vi "MotionMacro@CombineMotion__Parameter.vi"(1 "ParamterIn":string) -> (0 "ParamterOut":string)   [LabVIEW 2020]
panel:
  in  "AxisU":string(combo)
  in  "AxisZ":string(combo)
  in  "AxisY":string(combo)
  in  "AxisX":string(combo)
  in  "CombineMotor":string(combo)
  in  "Confirm":bool
  # "MotorMacro@CombineMotion $CombinName,$AxisX,$AxisY(,$AxisZ.....)"
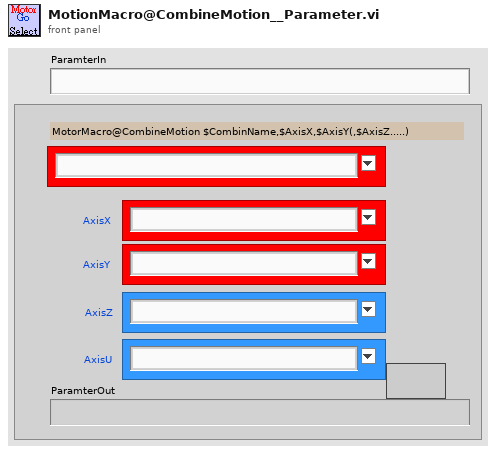
[diagram p1: front panel]
types:
  T1 = enum16{"Get", "Init", "Set", "Delete", "GetElement", "Inc", "Dec", "ReName", "Copy"}
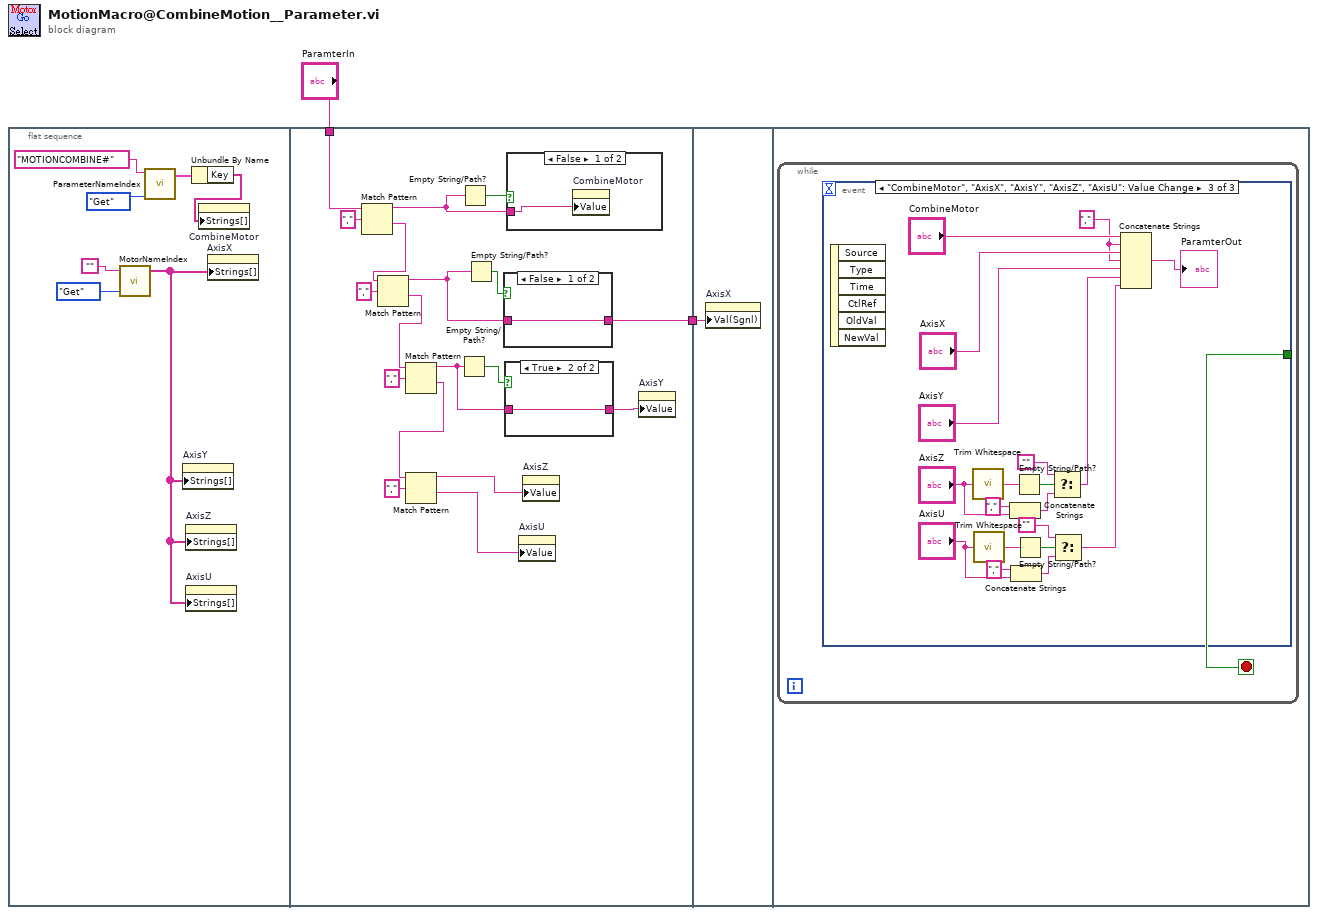
[diagram p0: block diagram]
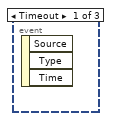
[diagram p5: hidden frame]
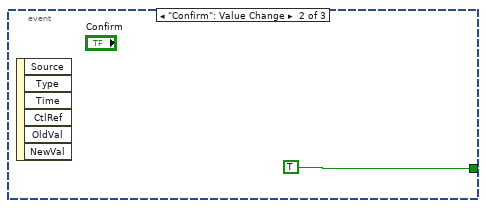
[diagram p6: hidden frame]
diagram:
  n1 = flat-sequence {
    tunnel: "ParamterIn" -> [w24]
    tunnel: [w25] -> w1
    tunnel: w1 -> [w33]
    frame #0 {
      n2 = call "MotorNameIndex.vi"("OP"=enum16{"Get", "Update", "Init"}."Get", "MotorName"="") -> ("MotorList"=w7:string[])  [unwired: 1 in, 2 out]
      n3 = call "ParameterNameIndex.vi"("OP"=T1."Get", "VariableSection"="MOTIONCOMBINE#" ("string")) -> ("SectionKeyValue"=w4:cluster{"Key":string[], "Value":string[]})  [unwired: 3 in, 6 out]
      n4 = property on="AxisY" class="CmbBox"("Strings[]"=w7) -> ()  [unwired: 2 in, 2 out]
      n5 = property on="AxisZ" class="CmbBox"("Strings[]"=w7) -> ()  [unwired: 2 in, 2 out]
      n6 = property on="AxisU" class="CmbBox"("Strings[]"=w7) -> ()  [unwired: 2 in, 2 out]
      n7 = Unbundle By Name(w4) -> ("Key"=w3:string[])
      n8 = property on="CombineMotor" class="CmbBox"("Strings[]"=w3) -> ()  [unwired: 2 in, 2 out]
      n9 = property on="AxisX" class="CmbBox"("Strings[]"=w7) -> ()  [unwired: 2 in, 2 out]
    }
    frame #1 {
      n10 = Match Pattern(string=w24, regular expression="," ("search string")) -> (before substring=w22:string, after substring=w20:string)  [unwired: 1 in, 2 out]
      n11 = Match Pattern(string=w20, regular expression="," ("search string")) -> (before substring=w19:string, after substring=w17:string)  [unwired: 1 in, 2 out]
      n12 = Match Pattern(string=w17, regular expression="," ("search string")) -> (before substring=w14:string, after substring=w12:string)  [unwired: 1 in, 2 out]
      n13 = Match Pattern(string=w12, regular expression="," ("search string")) -> (before substring=w11:string, after substring=w10:string)  [unwired: 1 in, 2 out]
      n14 = Empty String/Path?(string/path=w14) -> (empty?=w16:bool)
      n15 = Empty String/Path?(string/path=w22) -> (empty?=w27:bool)
      n16 = Empty String/Path?(string/path=w19) -> (empty?=w26:bool)
      n17 = case shown="False" w26 {
        tunnel: [w30 w31] -> w25
        tunnel: w19 -> [w30 w31]
        frame False {
        }
        frame True {
        }
      }
      n18 = case shown="True" w16 {
        tunnel: [w28 w29] -> w15
        tunnel: w14 -> [w28 w29]
        frame False {
        }
        frame True {
        }
      }
      n19 = case shown="False" w27 {
        tunnel: w22 -> [w32 _]
        frame False {
          n20 = property on="CombineMotor" class="CmbBox"("Value"=w32) -> ()  [unwired: 2 in, 2 out]
        }
        frame True {
        }
      }
      n21 = property on="AxisU" class="CmbBox"("Value"=w10) -> ()  [unwired: 2 in, 2 out]
      n22 = property on="AxisZ" class="CmbBox"("Value"=w11) -> ()  [unwired: 2 in, 2 out]
      n23 = property on="AxisY" class="CmbBox"("Value"=w15) -> ()  [unwired: 2 in, 2 out]
    }
    frame #2 {
      n24 = property on="AxisX" class="CmbBox"("Val(Sgnl)"=w33) -> ()  [unwired: 2 in, 2 out]
    }
    frame #3 {
      n25 = while {
        stop <- w34 stop-if-true
        n26 = event shown="[2] \"CombineMotor\", \"AxisX\", \"AxisY\", \"AxisZ\", \"AxisU\": Value Change" {
          selector: _ -> [_ _ _]
          dyn-events: _ -> [_ _ _]
          timeout: _ -> [_ _ _]
          tunnel: [_ TRUE _] -> w34
          event Timeout {
            n27 = event-data() -> ()  [unwired: 1 in, 3 out]
          }
          event "Confirm": Value Change {
            n28 = event-data() -> ()  [unwired: 1 in, 6 out]
          }
          event "CombineMotor", "AxisX", "AxisY", "AxisZ", "AxisU": Value Change {
            w50 = "," ("string")
            n29 = event-data() -> ()  [unwired: 1 in, 6 out]
            n30 = call <vilib>:"Trim Whitespace.vi"("string"="AxisZ") -> ("trimmed string"=w49:string)  [unwired: 1 in]
            n31 = call <vilib>:"Trim Whitespace.vi"("string"="AxisU") -> ("trimmed string"=w38:string)  [unwired: 1 in]
            n32 = Concatenate Strings("," ("string"), "AxisZ") -> (w44:string)
            n33 = Concatenate Strings("," ("string"), "AxisU") -> (w42:string)
            n34 = Empty String/Path?(string/path=w49) -> (empty?=w48:bool)
            n35 = Empty String/Path?(string/path=w38) -> (empty?=w39:bool)
            n36 = Select(t="", s=w48, f=w44) -> (s? t:f=w43:string)
            n37 = Select(t="", s=w39, f=w42) -> (s? t:f=w36:string)
            n38 = Concatenate Strings("CombineMotor", w50, "AxisX", w50, "AxisY", w43, w36) -> (→"ParamterOut":string)
          }
        }
      }
    }
  }
